vi "Initialize-object-wrapper-example.vi"(8 "error in (no error)":errorcluster) -> (0 "error out":errorcluster, 3 "Errors out":T1)   [LabVIEW 2013, in "Error-handling.lvlib" / "Errors.lvclass"]
uses:
  Errors.lvclass
  Object-reference.ctl
  Settings.ctl
  Languages.ctl
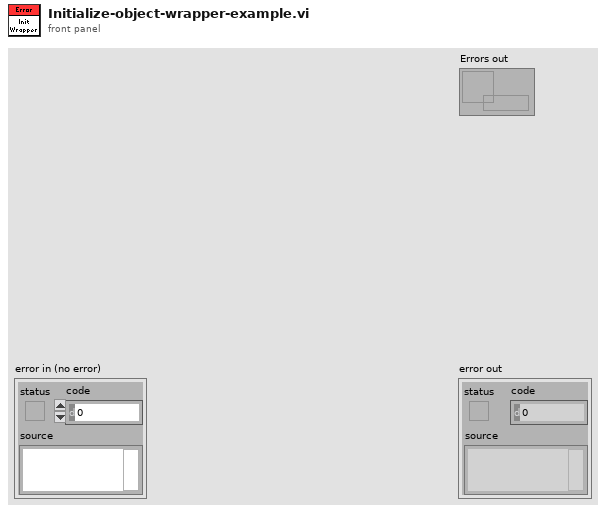
[diagram p1: front panel]
types:
  T1 = typedef "Error-handling.lvlib/Errors.lvclass/Object-reference.ctl" = refnum<data-value>
  T2 = typedef "Error-handling.lvlib/Errors.lvclass/Settings.ctl" = cluster{"Language":T3, "Display error dialog":bool, "Write log to file":bool, "Stream to log file":bool, "Overwrite existing log":bool, "Max log size":i32, "Max number of log files":i32}
  T3 = typedef "Error-handling.lvlib/Errors.lvclass/Languages.ctl" = enum16{"English"}
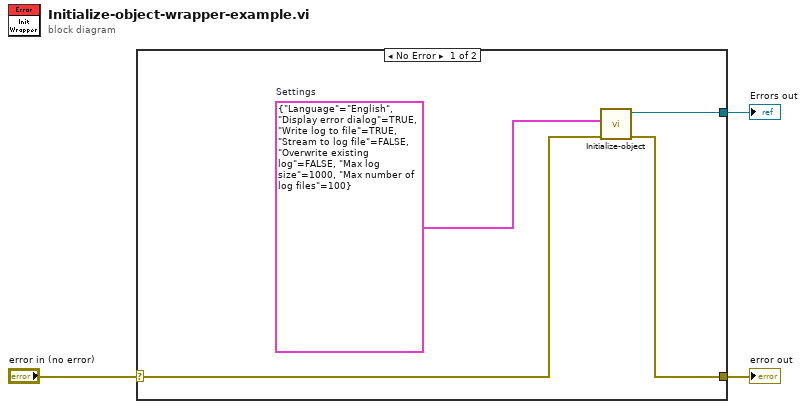
[diagram p0: block diagram]
diagram:
  n1 = case shown="No Error" "error in (no error)" {
    selector: "error in (no error)" -> [w5 w8]
    tunnel: [w6 w8] -> w2
    tunnel: [w7 _] -> w1
    frame No Error {
      w4 = T2 {"Language"=enum."English", "Display error dialog"=TRUE, "Write log to file"=TRUE, "Stream to log file"=FALSE, "Overwrite existing log"=FALSE, "Max log size"=1000, "Max number of log files"=100}  # Settings
      n2 = call "Initialize-object.vi"("error in (no error)"=w5, "Settings"=w4) -> ("error out"=w6:errorcluster, "Errors out"=w7:T1)  [unwired: 8 in]
    }
    frame Error {
    }
  }
  "error out" <- w2
  "Errors out" <- w1
